vi "close client handle.vi"(8 "error in (no error)":errorcluster, 11 "Oauth2 in":refnum<class "Oauth2.lvclass">) -> (0 "error out":errorcluster, 3 "Oauth2 out":refnum<class "Oauth2.lvclass">)   [LabVIEW 2020, in "Oauth2.lvclass"]
uses:
  Oauth2.lvclass
  Oauth2.lvclass/Oauth2.ctl
  OauthClient/OAuthClient.lvclass
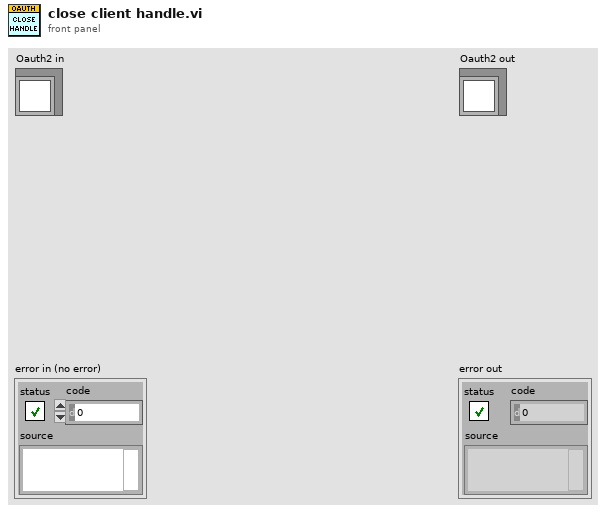
[diagram p1: front panel]
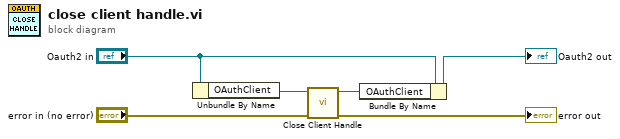
[diagram p0: block diagram]
diagram:
  n1 = Unbundle By Name("Oauth2 in") -> ("OAuthClient"=w2:refnum<class "OAuthClient.lvclass">)
  n2 = call-dynamic "Close Client Handle.vi"("error in (no error)"="error in (no error)", "OAuthClient in"=w2) -> ("error out"=→"error out":errorcluster, "OAuthClient out"=w1:refnum<class "OAuthClient.lvclass">)  [unwired: 8 in]
  n3 = Bundle By Name(cluster="Oauth2 in", "OAuthClient"=w1) -> (→"Oauth2 out":refnum<class "Oauth2.lvclass">)
